vi "QuickShoot.vi"() -> ()   [LabVIEW 2012]
uses:
  State_Machine_Enum.ctl
  Robot Global Data.vi
panel:
  in  "MinWait":u32
  in  "PullBackTolerenceMaxPercentDifference":dbl=0.1
  in  "FireTolerenceRPM 2":dbl=5.0
  in  "PullBackTolerence":dbl=50.0
  in  "FireTolerenceRPM":dbl=20.0
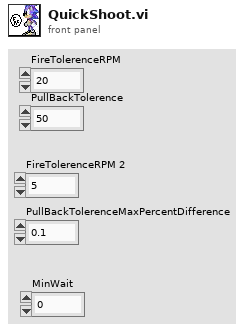
[diagram p1: front panel]
types:
  T1 = typedef "State_Machine_Enum.ctl" = enum16{"Idle", "Start", "Do", "Stop", "Init"}
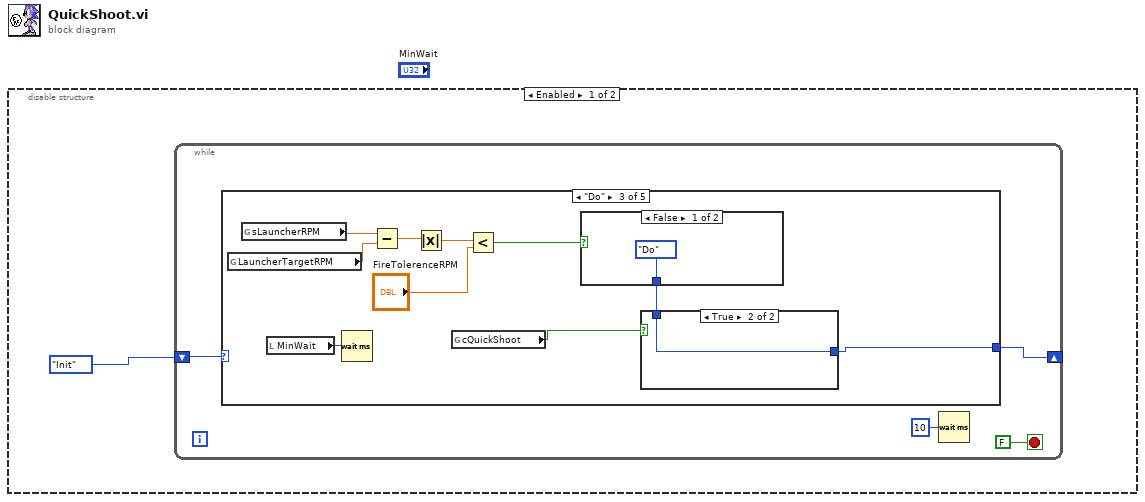
[diagram p0: block diagram]
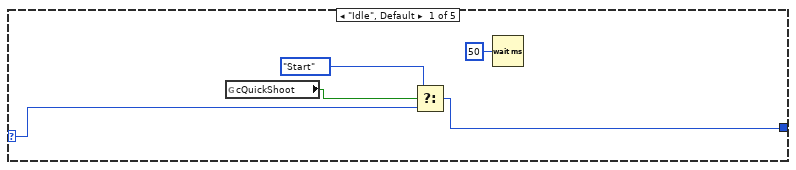
[diagram p2: hidden frame]
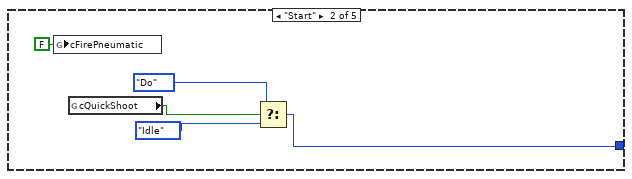
[diagram p3: hidden frame]
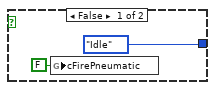
[diagram p4: hidden frame]
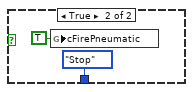
[diagram p5: hidden frame]
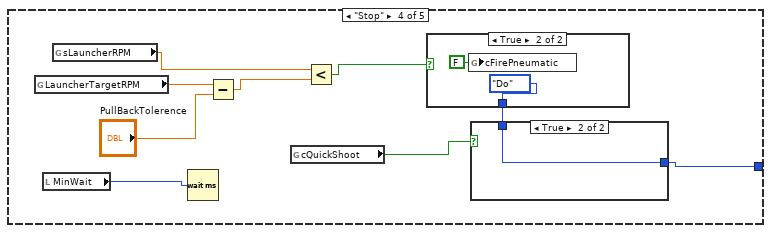
[diagram p6: hidden frame]
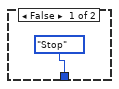
[diagram p7: hidden frame]
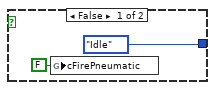
[diagram p8: hidden frame]
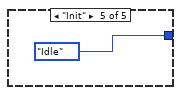
[diagram p9: hidden frame]
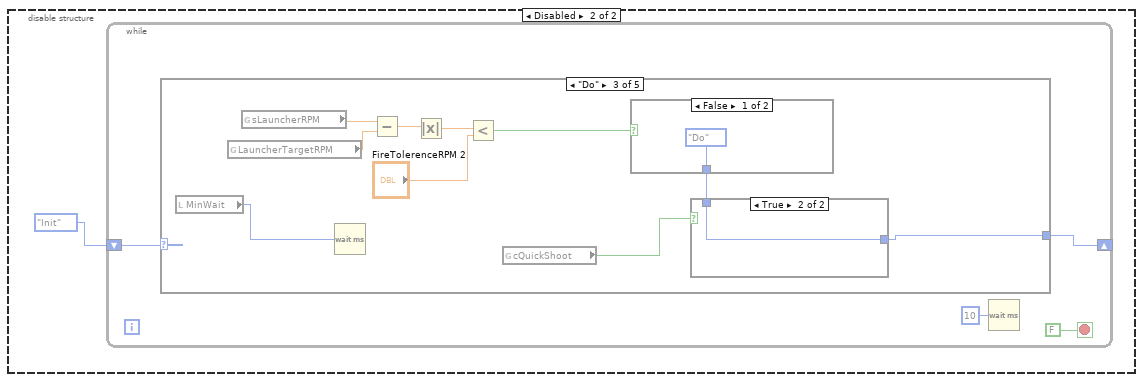
[diagram p10: hidden frame]
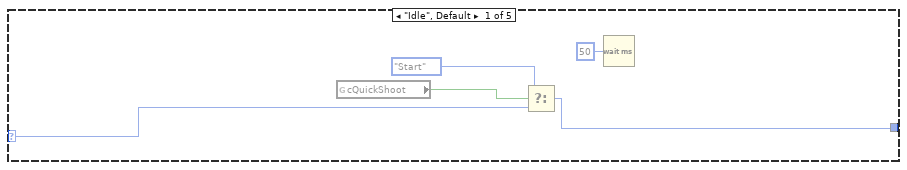
[diagram p11: hidden frame]
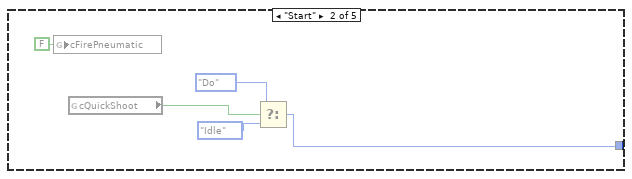
[diagram p12: hidden frame]
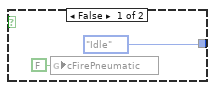
[diagram p13: hidden frame]
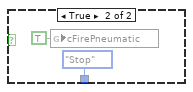
[diagram p14: hidden frame]
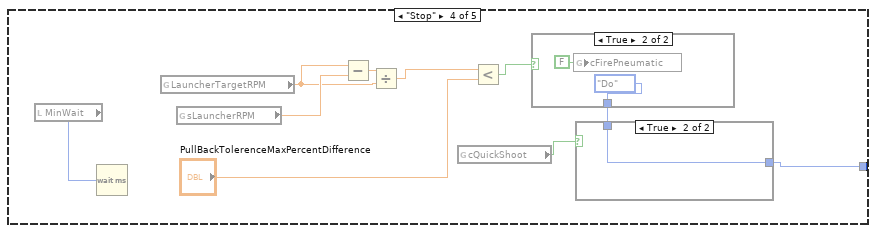
[diagram p15: hidden frame]
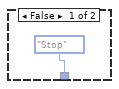
[diagram p16: hidden frame]
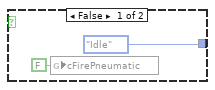
[diagram p17: hidden frame]
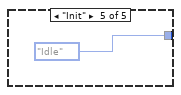
[diagram p18: hidden frame]
diagram:
  n1 = disable-structure shown="Enabled" {
    frame Enabled {
      n2 = while {
        shift-right: [w3] -> _
        shift-left: State_Machine_Enum."Init" ("State") -> [w4]
        stop <- FALSE stop-if-true
        n3 = case shown="\"Do\"" w4 {
          selector: w4 -> [w10 _ _ _ _]
          tunnel: [w9 w13 w17 w40 State_Machine_Enum."Idle" ("State")] -> w3
          frame "Idle", Default {
            n4 = global read "Robot Global Data.vi" "cQuickShoot"() -> (w8:bool)
            n5 = Select(t=State_Machine_Enum."Start", s=w8, f=w10) -> (s? t:f=w9:T1)
            n6 = Wait (ms)(milliseconds to wait=u32 50) -> ()  [unwired: 1 out]
          }
          frame "Start" {
            n7 = global write "Robot Global Data.vi" "cFirePneumatic"(FALSE ("cFirePneumatic")) -> ()
            n8 = global read "Robot Global Data.vi" "cQuickShoot"() -> (w15:bool)
            n9 = Select(t=State_Machine_Enum."Do", s=w15, f=State_Machine_Enum."Idle") -> (s? t:f=w13:T1)
          }
          frame "Do" {
            n10 = global read "Robot Global Data.vi" "LauncherTargetRPM"() -> (w24:dbl)
            n11 = global read "Robot Global Data.vi" "sLauncherRPM"() -> (w25:dbl)
            n12 = local read "MinWait"() -> (w16:u32)
            n13 = Wait (ms)(milliseconds to wait=w16) -> ()  [unwired: 1 out]
            n14 = Subtract(x=w25, y=w24) -> (x-y=w23:dbl)
            n15 = Absolute Value(x=w23) -> (abs(x)=w21:dbl)
            n16 = global read "Robot Global Data.vi" "cQuickShoot"() -> (w19:bool)
            n17 = Less?(x=w21, y="FireTolerenceRPM") -> (x < y?=w20:bool)
            n18 = case shown="False" w20 {
              tunnel: [State_Machine_Enum."Do" ("t") State_Machine_Enum."Stop" ("t")] -> w18
              frame False {
              }
              frame True {
                n19 = global write "Robot Global Data.vi" "cFirePneumatic"(TRUE ("cFirePneumatic")) -> ()
              }
            }
            n20 = case shown="True" w19 {
              tunnel: [State_Machine_Enum."Idle" ("f") w28] -> w17
              tunnel: w18 -> [_ w28]
              frame False {
                n21 = global write "Robot Global Data.vi" "cFirePneumatic"(FALSE ("cFirePneumatic")) -> ()
              }
              frame True {
              }
            }
          }
          frame "Stop" {
            n22 = global read "Robot Global Data.vi" "LauncherTargetRPM"() -> (w38:dbl)
            n23 = local read "MinWait"() -> (w32:u32)
            n24 = global read "Robot Global Data.vi" "sLauncherRPM"() -> (w36:dbl)
            n25 = Wait (ms)(milliseconds to wait=w32) -> ()  [unwired: 1 out]
            n26 = Subtract(x=w38, y="PullBackTolerence") -> (x-y=w35:dbl)
            n27 = global read "Robot Global Data.vi" "cQuickShoot"() -> (w39:bool)
            n28 = Less?(x=w36, y=w35) -> (x < y?=w34:bool)
            n29 = case shown="True" w34 {
              tunnel: [State_Machine_Enum."Stop" ("t") State_Machine_Enum."Do" ("t")] -> w33
              frame False {
              }
              frame True {
                n30 = global write "Robot Global Data.vi" "cFirePneumatic"(FALSE ("cFirePneumatic")) -> ()
              }
            }
            n31 = case shown="True" w39 {
              tunnel: [State_Machine_Enum."Idle" ("f") w46] -> w40
              tunnel: w33 -> [_ w46]
              frame False {
                n32 = global write "Robot Global Data.vi" "cFirePneumatic"(FALSE ("cFirePneumatic")) -> ()
              }
              frame True {
              }
            }
          }
          frame "Init" {
          }
        }
        n33 = Wait (ms)(milliseconds to wait=u32 10) -> ()  [unwired: 1 out]
      }
    }
    frame Disabled {
      n34 = while {
        shift-right: [w50] -> _
        shift-left: State_Machine_Enum."Init" ("State") -> [w51]
        stop <- FALSE stop-if-true
        n35 = case shown="\"Do\"" w51 {
          selector: w51 -> [w57 _ _ _ _]
          tunnel: [w56 w60 w69 w88 State_Machine_Enum."Idle" ("State")] -> w50
          frame "Idle", Default {
            n36 = global read "Robot Global Data.vi" "cQuickShoot"() -> (w55:bool)
            n37 = Select(t=State_Machine_Enum."Start", s=w55, f=w57) -> (s? t:f=w56:T1)
            n38 = Wait (ms)(milliseconds to wait=u32 50) -> ()  [unwired: 1 out]
          }
          frame "Start" {
            n39 = global write "Robot Global Data.vi" "cFirePneumatic"(FALSE ("cFirePneumatic")) -> ()
            n40 = global read "Robot Global Data.vi" "cQuickShoot"() -> (w62:bool)
            n41 = Select(t=State_Machine_Enum."Do", s=w62, f=State_Machine_Enum."Idle") -> (s? t:f=w60:T1)
          }
          frame "Do" {
            n42 = local read "MinWait"() -> (w63:u32)
            n43 = global read "Robot Global Data.vi" "LauncherTargetRPM"() -> (w67:dbl)
            n44 = global read "Robot Global Data.vi" "sLauncherRPM"() -> (w68:dbl)
            n45 = Wait (ms)(milliseconds to wait=w63) -> ()  [unwired: 1 out]
            n46 = Subtract(x=w68, y=w67) -> (x-y=w66:dbl)
            n47 = Absolute Value(x=w66) -> (abs(x)=w64:dbl)
            n48 = Less?(x=w64, y="FireTolerenceRPM 2") -> (x < y?=w72:bool)
            n49 = global read "Robot Global Data.vi" "cQuickShoot"() -> (w71:bool)
            n50 = case shown="False" w72 {
              tunnel: [State_Machine_Enum."Do" ("t") State_Machine_Enum."Stop" ("t")] -> w70
              frame False {
              }
              frame True {
                n51 = global write "Robot Global Data.vi" "cFirePneumatic"(TRUE ("cFirePneumatic")) -> ()
              }
            }
            n52 = case shown="True" w71 {
              tunnel: [State_Machine_Enum."Idle" ("f") w75] -> w69
              tunnel: w70 -> [_ w75]
              frame False {
                n53 = global write "Robot Global Data.vi" "cFirePneumatic"(FALSE ("cFirePneumatic")) -> ()
              }
              frame True {
              }
            }
          }
          frame "Stop" {
            n54 = local read "MinWait"() -> (w79:u32)
            n55 = Wait (ms)(milliseconds to wait=w79) -> ()  [unwired: 1 out]
            n56 = global read "Robot Global Data.vi" "LauncherTargetRPM"() -> (w80:dbl)
            n57 = global read "Robot Global Data.vi" "sLauncherRPM"() -> (w82:dbl)
            n58 = Subtract(x=w80, y=w82) -> (x-y=w81:dbl)
            n59 = Divide(x=w81, y=w80) -> (x/y=w84:dbl)
            n60 = global read "Robot Global Data.vi" "cQuickShoot"() -> (w87:bool)
            n61 = Less?(x=w84, y="PullBackTolerenceMaxPercentDifference") -> (x < y?=w86:bool)
            n62 = case shown="True" w86 {
              tunnel: [State_Machine_Enum."Stop" ("t") State_Machine_Enum."Do" ("t")] -> w85
              frame False {
              }
              frame True {
                n63 = global write "Robot Global Data.vi" "cFirePneumatic"(FALSE ("cFirePneumatic")) -> ()
              }
            }
            n64 = case shown="True" w87 {
              tunnel: [State_Machine_Enum."Idle" ("f") w94] -> w88
              tunnel: w85 -> [_ w94]
              frame False {
                n65 = global write "Robot Global Data.vi" "cFirePneumatic"(FALSE ("cFirePneumatic")) -> ()
              }
              frame True {
              }
            }
          }
          frame "Init" {
          }
        }
        n66 = Wait (ms)(milliseconds to wait=u32 10) -> ()  [unwired: 1 out]
      }
    }
  }
